vi "AI Base Initialize.vi"(0 "OpenAI API URL":string caption="OpenAI API URL (e.g. OpenRouter, LM Studio)", 1 "Python venv path":path=path "C:/dev/gaoruhao/labview-ai", 5 "API Key":string, 9 "Python version":string, 11 "error in (no error)":errorcluster, 12 "Anaconda path":path=path "C:/ProgramData/miniforge3", 13 "conda env name":string="ai") -> (4 "Python Refnum out":refnum<k35>, 10 "Http Client Handle out":T1, 15 "error out":errorcluster)   [LabVIEW 2023, in "LabVIEW AI Base.lvlib"]
uses:
  LabVIEW AI Base.lvlib
  <vilib>/httpClient/ClientHandle.ctl
  <vilib>/Utility/error.llb/Trim Whitespace One-Sided.vi
  AI Base Globals.vi
  <vilib>/Python/Open Venv Python Session.vi
  <vilib>/Python/Open Anaconda Python Session.vi
  <vilib>/httpClient/LabVIEWHTTPClient.lvlib
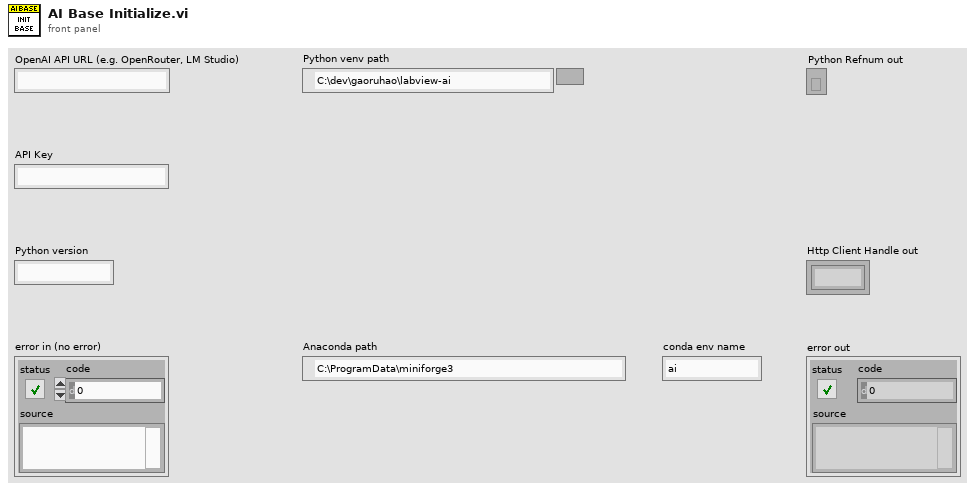
[diagram p1: front panel]
types:
  T1 = typedef "LabVIEWHTTPClient.lvlib/ClientHandle.ctl" = refnum<k1>
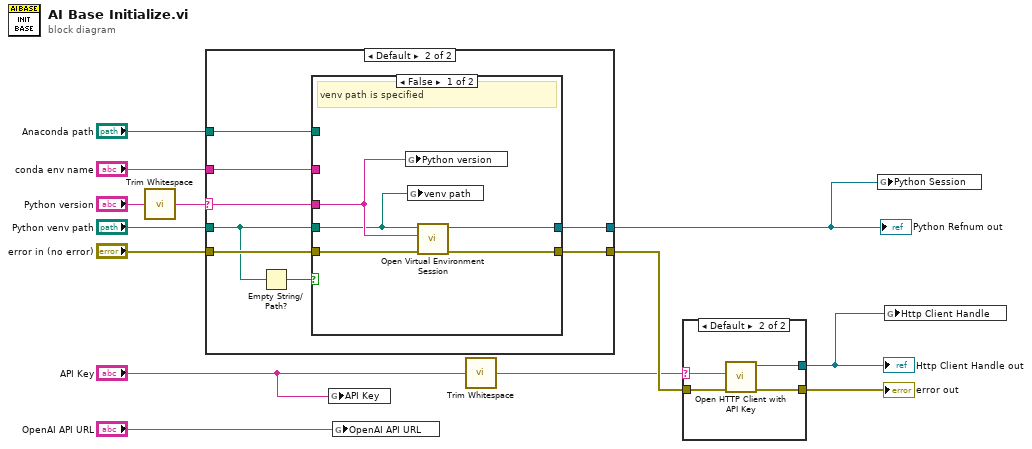
[diagram p0: block diagram]
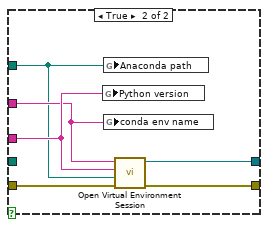
[diagram p4: hidden frame]
diagram:
  n1 = call <vilib>:"Trim Whitespace.vi"("string"="Python version") -> ("trimmed string"=w2:string)  [unwired: 1 in]
  n2 = case shown="Default" w2 {
    selector: w2 -> [_ w21]
    tunnel: [w14 w22] -> w13
    tunnel: "error in (no error)" -> [w14 w20]
    tunnel: "Python venv path" -> [_ w18]
    tunnel: "Anaconda path" -> [_ w17]
    tunnel: "conda env name" -> [_ w16]
    tunnel: [_ w15] -> w4
    frame "" {
    }
    frame Default {
      n3 = Empty String/Path?(string/path=w18) -> (empty?=w19:bool)
      n4 = case shown="False" w19 {
        tunnel: [w27 w33] -> w15
        tunnel: [w26 w32] -> w22
        tunnel: w21 -> [w25 w31]
        tunnel: w20 -> [w24 w30]
        tunnel: w18 -> [w23 _]
        tunnel: w17 -> [_ w28]
        tunnel: w16 -> [_ w29]
        frame False {
          # "venv path is specified"
          n5 = global write "AI Base Globals.vi" "Python version"(w25) -> ()
          n6 = global write "AI Base Globals.vi" "venv path"(w23) -> ()
          n7 = call-poly <vilib>:"Open Virtual Environment Session.vi"("error in (no error)"=w24, "Python version"=w25, "Env path"=w23) -> ("error out"=w26:errorcluster, "session out"=w27:refnum<k35>)  [unwired: 7 in]
        }
        frame True {
          n8 = global write "AI Base Globals.vi" "Python version"(w31) -> ()
          n9 = global write "AI Base Globals.vi" "Anaconda path"(w28) -> ()
          n10 = global write "AI Base Globals.vi" "conda env name"(w29) -> ()
          n11 = call-poly <vilib>:"Open Virtual Environment Session.vi"("error in (no error)"=w30, "Anaconda path"=w28, "Python version"=w31, "Env name"=w29) -> ("error out"=w32:errorcluster, "session out"=w33:refnum<k35>)  [unwired: 6 in]
        }
      }
    }
  }
  "Python Refnum out" <- w4
  n12 = global write "AI Base Globals.vi" "API Key"("API Key") -> ()
  n13 = global write "AI Base Globals.vi" "OpenAI API URL"("OpenAI API URL") -> ()
  n14 = call <vilib>:"Trim Whitespace.vi"("string"="API Key") -> ("trimmed string"=w1:string)  [unwired: 1 in]
  n15 = case shown="Default" w1 {
    selector: w1 -> [_ w36]
    tunnel: w13 -> [w34 w38]
    tunnel: [w34 w37] -> w12
    tunnel: [_ w35] -> w3
    frame "\u0000" {
    }
    frame Default {
      n16 = call "Open HTTP Client with API Key.vi"("error in"=w38, "API Key"=w36) -> ("error out"=w37:errorcluster, "Refnum out"=w35:T1)  [unwired: 8 in]
    }
  }
  "error out" <- w12
  "Http Client Handle out" <- w3
  n17 = global write "AI Base Globals.vi" "Python Session"(w4) -> ()
  n18 = global write "AI Base Globals.vi" "Http Client Handle"(w3) -> ()
